vi "Allocate En Face Array.vi"(9 "Number of B-Scans":u32, 10 "A-Scans Per B-Scan":u32, 11 ">> En Face Array >>":sgl[][](array[numeric])) -> (3 "Array":sgl[][](array[numeric]))   [LabVIEW 2015, in "Intensity Processing.lvclass"]
uses:
  Intensity/Intensity Processing.lvclass
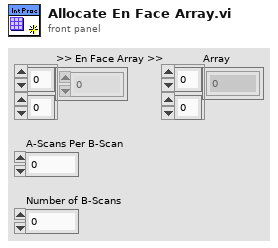
[diagram p1: front panel]
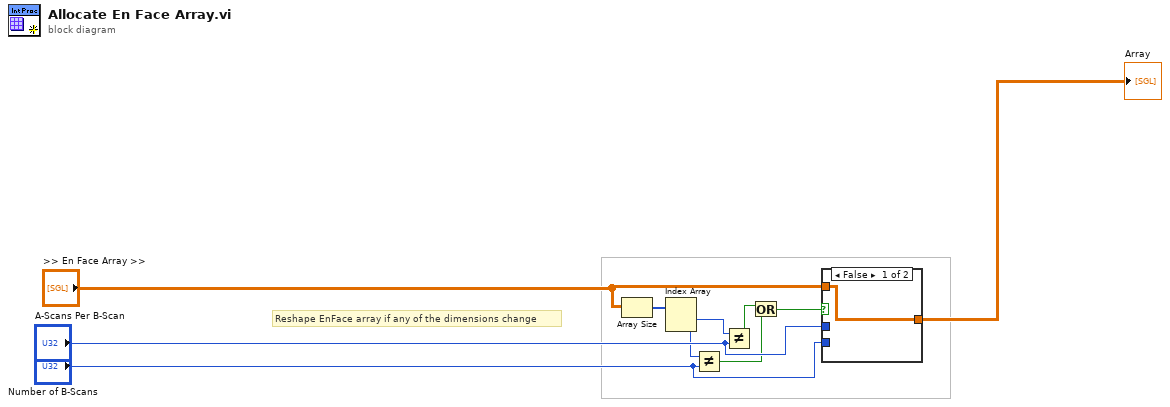
[diagram p0: block diagram]
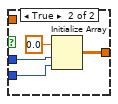
[diagram p2: hidden frame]
diagram:
  # "Reshape EnFace array if any of the dimensions change"
  n1 = Array Size(array=">> En Face Array >>") -> (size(s)=w2:i32[])
  n2 = Index Array(array=w2) -> (element #1=w4:i32, element #2=w3:i32)  [unwired: 2 in]
  n3 = Not Equal?(x=w3, y="Number of B-Scans") -> (x != y?=w6:bool)
  n4 = Not Equal?(x=w4, y="A-Scans Per B-Scan") -> (x != y?=w7:bool)
  n5 = Or(x=w7, y=w6) -> (x .or. y?=w5:bool)
  n6 = case shown="False" w5 {
    tunnel: "A-Scans Per B-Scan" -> [_ w14]
    tunnel: "Number of B-Scans" -> [_ w13]
    tunnel: [w11 w12] -> w8
    tunnel: ">> En Face Array >>" -> [w11 _]
    frame False {
    }
    frame True {
      n7 = Initialize Array(sgl 0.0 ("element"), w14, w13) -> (w12:sgl[][])
    }
  }
  "Array" <- w8
